vi "wait HOLD.vi"(8 "error in (no error)":errorcluster) -> (0 "error out":errorcluster)   [LabVIEW 2016]
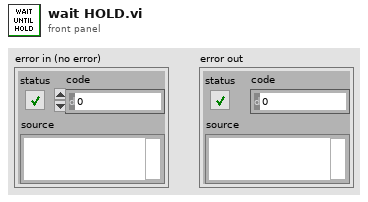
[diagram p1: front panel]
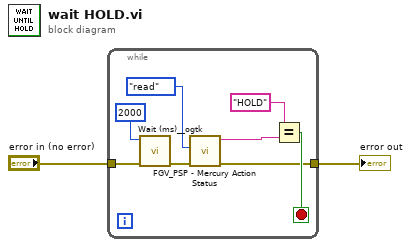
[diagram p0: block diagram]
diagram:
  n1 = while {
    tunnel: "error in (no error)" -> [w4]
    tunnel: [w8] -> w1
    stop <- w10 stop-if-true
    n2 = call <userlib>:"Wait (ms)__ogtk.vi"("error in (no error)"=w4, "milliseconds to wait"=u32 2000) -> ("error out"=w5:errorcluster)  [unwired: 8 in, 1 out]
    n3 = call "FGV_PSP - Mercury Action Status.vi"("error in"=w5, "Function"=enum16{"write", "read"}."read") -> ("error out"=w8:errorcluster, "Mercury Status 2"=w3:string)  [unwired: 4 in]
    n4 = Equal?(x="HOLD", y=w3) -> (x = y?=w10:bool)
  }
  "error out" <- w1
